vi "分割屏幕并获取指定块坐标.vi"(6 "位置":i32, 8 "error in (no error)":errorcluster caption="错误输入（无错误）", 9 "行数":i32, 10 "列数":i32, 11 "引用":refnum<vi>) -> (0 "error out":errorcluster caption="错误输出", 2 "指定块顶点":cluster{"左":i32, "上":i32}, 3 "引用输出":refnum<vi>)   [LabVIEW 8.6, in "窗口操作.lvlib"]
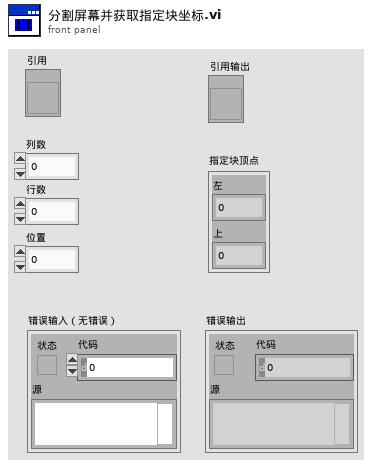
[diagram p1: front panel]
types:
  T1 = typedef "LVRectTypeDef.ctl" = cluster{"Left":i16, "Top":i16, "Right":i16, "Bottom":i16}
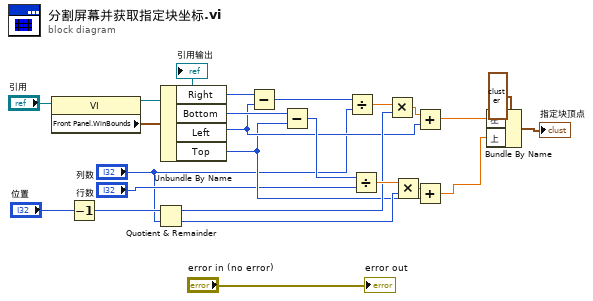
[diagram p0: block diagram]
diagram:
  n1 = property class="VI"(reference="引用") -> (reference out=→"引用输出":refnum<vi>, "Front Panel.WinBounds"=w24:T1)  [unwired: 1 in, 1 out]
  n2 = Decrement(x="位置") -> (x-1=w10:i32)
  n3 = Quotient & Remainder(x=w10, y="列数") -> (x-y*floor(x/y)=w16:i32, floor(x/y)=w15:i32)
  n4 = Unbundle By Name(w24) -> ("Right"=w23:i16, "Bottom"=w22:i16, "Left"=w12:i16, "Top"=w11:i16)
  n5 = Subtract(x=w23, y=w12) -> (x-y=w21:i16)
  n6 = Subtract(x=w22, y=w11) -> (x-y=w20:i16)
  n7 = Divide(x=w21, y="列数") -> (x/y=w18:dbl)
  n8 = Divide(x=w20, y="行数") -> (x/y=w17:dbl)
  n9 = Multiply(x=w18, y=w16) -> (x*y=w14:dbl)
  n10 = Multiply(x=w17, y=w15) -> (x*y=w13:dbl)
  n11 = Add(x=w14, y=w12) -> (x+y=w5:dbl)
  n12 = Add(x=w13, y=w11) -> (x+y=w4:dbl)
  n13 = Bundle By Name(cluster=cluster{"左":i32, "上":i32} ? ("指定块顶点"), "左"=w5, "上"=w4) -> (→"指定块顶点":cluster{"左":i32, "上":i32})
  "error out" <- "error in (no error)"
